vi "Pre Launch Init.vi"(11 "Vehicle Position Simulation in":refnum<class "Vehicle Position Simulation.lvclass">) -> (0 "error out":errorcluster, 3 "Vehicle Position Simulation out":refnum<class "Vehicle Position Simulation.lvclass">)   [LabVIEW 2019, in "Vehicle Position Simulation.lvlib" / "Vehicle Position Simulation.lvclass"]
doc: "(<B>Filename</B>: Actor Framework.lvlib:Actor.lvclass:Pre Launch Init.vi)\n\nDefines behavior that occurs after the Launch Nested Actor method is invoked but before the actor's Actor Core method begins running.\n\nBy default, this method does nothing. A descendant class may override it to define behavior."
uses:
  Vehicle Position Simulation.lvclass
  Vehicle Position Simulation.lvclass/Vehicle Position Simulation.ctl
  Abstract Vehicle Position Interface/Abstract Vehicle Position Interface/Vehicle Position Interface.lvclass
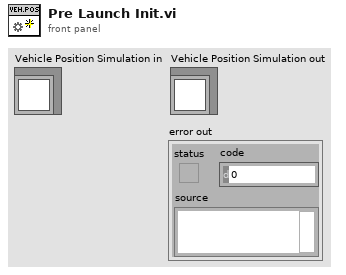
[diagram p1: front panel]
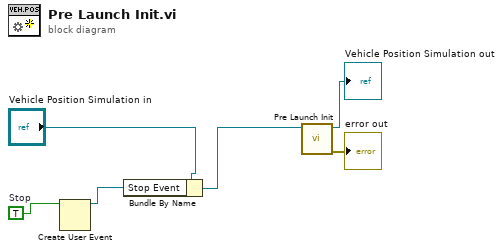
[diagram p0: block diagram]
diagram:
  w4 = TRUE  # Stop
  n1 = Create User Event(user event datatype=w4) -> (user event=w3:refnum<user-event>)  [unwired: 1 in, 1 out]
  n2 = Bundle By Name(cluster="Vehicle Position Simulation in", "Stop Event"=w3) -> (w1:refnum<class "Vehicle Position Simulation.lvclass">)
  n3 = call-parent "Pre Launch Init.vi"("Actor in"=w1) -> ("error out"=→"error out":errorcluster, "Actor out"=→"Vehicle Position Simulation out":refnum<class "Vehicle Position Simulation.lvclass">)  [unwired: 9 in]
